vi "Create Impl Class.vi"(0 "User Server Library in":refnum<vi>, 1 "RPC Method Parameters":T1[](array[typedef]), 7 ">>Application instance>> in":refnum<vi>, 11 "error in (no error)":errorcluster) -> (4 "User Server Library out":refnum<vi>, 8 ">>Application instance>> out":refnum<vi>, 10 "Service Impl class out":refnum<vi>, 15 "error IO":errorcluster)   [LabVIEW 2019, in "gRPC Template Creation Utility.lvlib"]
uses:
  gRPC Template Creation Utility.lvlib
  TypeDefs/RPC Method Parameters.ctl
  ServiceConstants.ctl
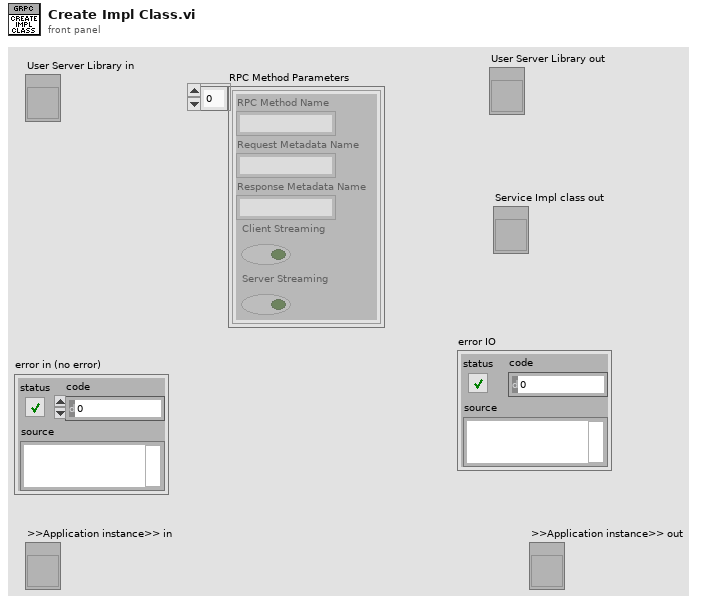
[diagram p1: front panel]
types:
  T1 = typedef "gRPC Template Creation Utility.lvlib/RPC Method Parameters.ctl" = cluster{"RPC Method Name":string, "Request Metadata Name":string, "Response Metadata Name":string, "Client Streaming":bool, "Server Streaming":bool}
  T2 = typedef "gRPC Template Creation Utility.lvlib/ServiceConstants.ctl" = enum16{"Stub", "Impl", "Usercode_server", "Generated_server", "RPC Service", "RPC Method package_service_method", "ServiceClass out", "ServiceClass in", "RPC Method"}
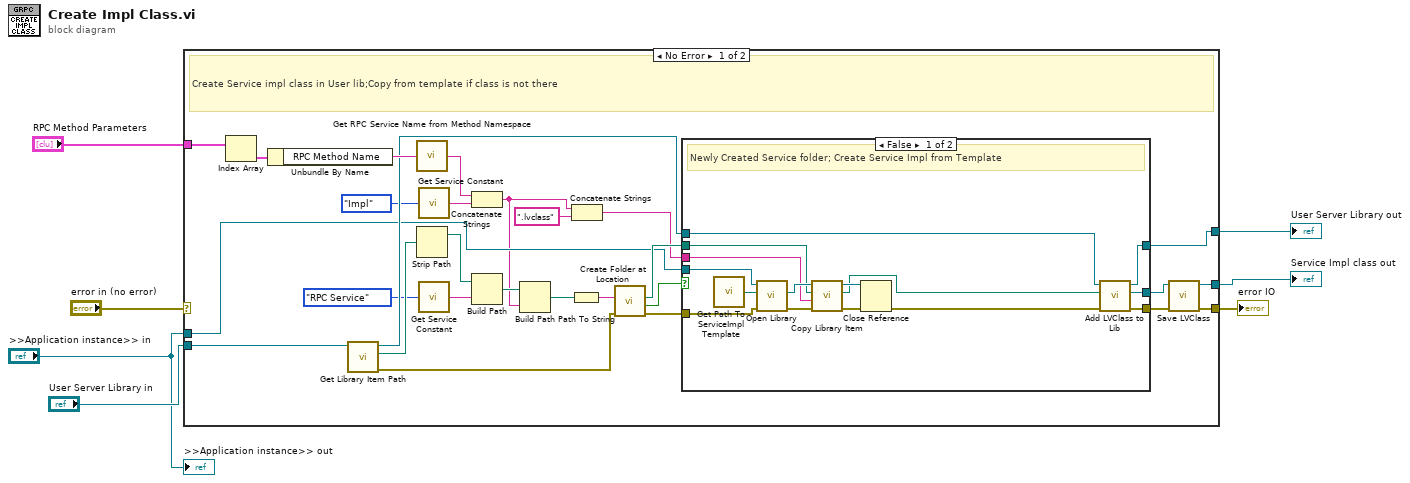
[diagram p0: block diagram]
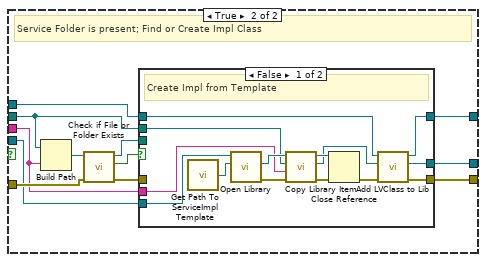
[diagram p2: hidden frame]
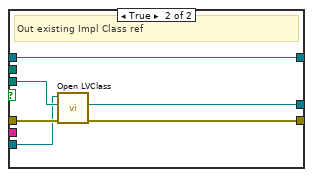
[diagram p3: hidden frame]
diagram:
  n1 = case shown="No Error" "error in (no error)" {
    selector: "error in (no error)" -> [_ w84]
    tunnel: "RPC Method Parameters" -> [w30 _]
    tunnel: "User Server Library in" -> [w27 w83]
    tunnel: [w26 _] -> w5
    tunnel: [w25 w84] -> w6
    tunnel: [w12 w83] -> w7
    tunnel: ">>Application instance>> in" -> [w11 _]
    frame No Error {
      # "Create Service impl class in User lib;Copy from template if class is not there"
      n2 = Index Array(array=w30) -> (element=w29:T1)  [unwired: 1 in]
      n3 = Unbundle By Name(w29) -> ("RPC Method Name"=w28:string)
      n4 = call "Get Library Item Path.vi"("Library"=w27) -> ("error out"=w32:errorcluster, "Path"=w35:path, "Library"=w21:refnum<vi>)  [unwired: 8 in]
      n5 = call "Get RPC Service Name from Method Namespace.vi"("RPC Method Name"=w28) -> ("RPC Service Name"=w31:string)
      n6 = Strip Path(path=w35) -> (stripped path=w34:path)  [unwired: 1 out]
      n7 = call "Get Service Constant.vi"("Service Constant Strings"=ServiceConstants."Impl") -> ("String Value"=w14:string)
      n8 = call "Get Service Constant.vi"("Service Constant Strings"=ServiceConstants."RPC Service") -> ("String Value"=w17:string)
      n9 = Concatenate Strings(w31, w14) -> (w10:string)
      n10 = Build Path(base path=w34, name or relative path=w17) -> (appended path=w15:path)
      n11 = Build Path(base path=w15, name or relative path=w10) -> (appended path=w13:path)
      n12 = Path To String(path=w13) -> (string=w33:string)
      n13 = Concatenate Strings(w10, ".lvclass" ("string")) -> (w19:string)
      n14 = call "Create Folder at Location.vi"("Error In"=w32, "Path"=w33) -> ("Error Out"=w23:errorcluster, "Already Exists ?"=w24:bool, "Full path out"=w22:path)  [unwired: 7 in]
      n15 = case shown="False" w24 {
        tunnel: w23 -> [w47 w61]
        tunnel: w22 -> [w44 w52]
        tunnel: w21 -> [w42 w55]
        tunnel: [w40 w57] -> w9
        tunnel: [w39 w56] -> w8
        tunnel: w19 -> [w38 w53]
        tunnel: [w37 w54] -> w12
        tunnel: w11 -> [w36 w51]
        frame False {
          # "Newly Created Service folder; Create Service Impl from Template"
          n16 = call "Get Path To ServiceImpl Template.vi"() -> ("appended path"=w46:path)
          n17 = call "Open Library.vi"("error in (no error)"=w47, "Full Path"=w46, "Application in"=w36) -> ("error out"=w43:errorcluster, "Library out"=w45:refnum<vi>)  [unwired: 6 in, 1 out]
          n18 = call "Copy Library Item.vi"("error in (no error)"=w43, "Copy Name"=w38, "Copy location"=w44, "Library in"=w45) -> ("error out"=w50:errorcluster, "New Lib Path"=w41:path, "Library out"=w49:refnum<vi>)  [unwired: 5 in]
          n19 = Close Reference(reference=w49, error in (no error)=w50) -> (error out=w48:errorcluster)
          n20 = call "Add LVClass to Lib.vi"("error in (no error)"=w48, "LVClass Path in"=w41, "Library in"=w42) -> ("error out"=w39:errorcluster, "LVClassLibrary out"=w40:refnum<vi>, "Library out"=w37:refnum<vi>)  [unwired: 6 in]
        }
        frame True {
          # "Service Folder is present; Find or Create Impl Class"
          n21 = Build Path(base path=w52, name or relative path=w53) -> (appended path=w62:path)
          n22 = call <vilib>:"Check if File or Folder Exists.vi"("error in (no error)"=w61, "path"=w62) -> ("error out"=w58:errorcluster, "file or folder exists?"=w60:bool, "dup path"=w59:path)  [unwired: 7 in]
          n23 = case shown="False" w60 {
            tunnel: w59 -> [_ w82]
            tunnel: w58 -> [_ w80]
            tunnel: [w66 w81] -> w57
            tunnel: [w68 w79] -> w56
            tunnel: w55 -> [w69 w78]
            tunnel: [w67 w78] -> w54
            tunnel: w53 -> [w65 _]
            tunnel: w52 -> [w64 _]
            tunnel: w51 -> [w63 w77]
            frame False {
              # "Create Impl from Template"
              n24 = call "Get Path To ServiceImpl Template.vi"() -> ("appended path"=w73:path)
              n25 = call "Open Library.vi"("Full Path"=w73, "Application in"=w63) -> ("error out"=w71:errorcluster, "Library out"=w72:refnum<vi>)  [unwired: 7 in, 1 out]
              n26 = call "Copy Library Item.vi"("error in (no error)"=w71, "Copy Name"=w65, "Copy location"=w64, "Library in"=w72) -> ("error out"=w76:errorcluster, "New Lib Path"=w70:path, "Library out"=w75:refnum<vi>)  [unwired: 5 in]
              n27 = Close Reference(reference=w75, error in (no error)=w76) -> (error out=w74:errorcluster)
              n28 = call "Add LVClass to Lib.vi"("error in (no error)"=w74, "LVClass Path in"=w70, "Library in"=w69) -> ("error out"=w68:errorcluster, "LVClassLibrary out"=w66:refnum<vi>, "Library out"=w67:refnum<vi>)  [unwired: 6 in]
            }
            frame True {
              # "Out existing Impl Class ref"
              n29 = call "Open LVClass.vi"("error in (no error)"=w80, "Full Path"=w82, "Application reference in"=w77) -> ("error out"=w79:errorcluster, "LVClass out"=w81:refnum<vi>)  [unwired: 6 in, 1 out]
            }
          }
        }
      }
      n30 = call "Save LVClass.vi"("error in (no error)"=w8, "LVClassLibrary in"=w9) -> ("error out"=w25:errorcluster, "LVClassLibrary out"=w26:refnum<vi>)  [unwired: 8 in]
    }
    frame Error {
    }
  }
  "User Server Library out" <- w7
  "error IO" <- w6
  "Service Impl class out" <- w5
  ">>Application instance>> out" <- ">>Application instance>> in"
